vi "3.1.vi"(8 "error in (no error)":errorcluster, 10 "String":string) -> (0 "error out":errorcluster, 2 "Numeric":i32)   [LabVIEW 2017]
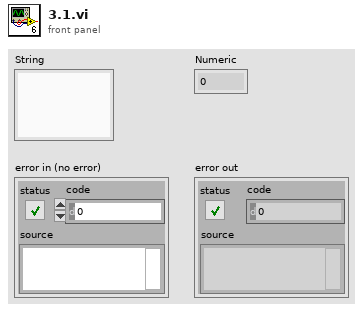
[diagram p1: front panel]
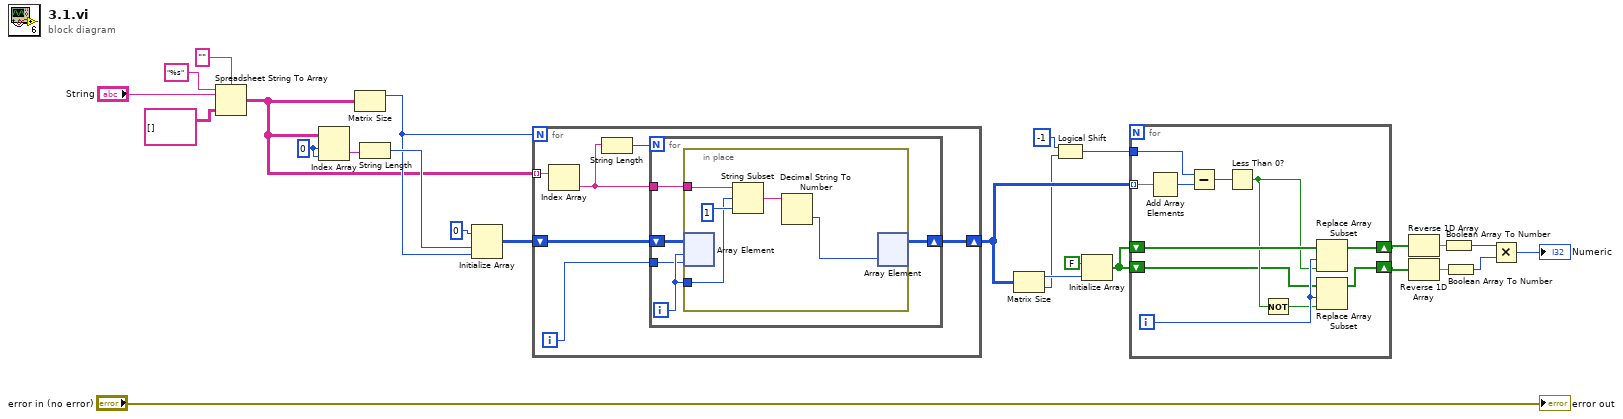
[diagram p0: block diagram]
diagram:
  w22 = 0 ("index (row)")
  n1 = Spreadsheet String To Array(delimiter (Tab)="", format string="%s", spreadsheet string="String", array type (2D Dbl)=string[][] []) -> (array=w15:string[][])
  n2 = Index Array(array=w15, index (row)=w22, index (col)=w22) -> (element=w21:string)
  n3 = Matrix Size(0:w15) -> (1:w16:i32)  [unwired: 1 out]
  n4 = String Length(string=w21) -> (length=w18:i32)
  n5 = Initialize Array(0 ("element"), w18, w16) -> (w17:i32[][])
  n6 = for {
    N: w16 -> [_]
    tunnel: w15 -> [w30] mode=indexing
    shift-right: [w27] -> w13
    shift-left: w17 -> [w32]
    i -> [w31]
    n7 = Index Array(array=w30) -> (element=w29:string)  [unwired: 1 in]
    n8 = String Length(string=w29) -> (length=w28:i32)
    n9 = for {
      N: w28 -> [_]
      shift-right: [w35] -> w27
      shift-left: w32 -> [w37]
      tunnel: w31 -> [w33]
      tunnel: w29 -> [w36]
      i -> [w34]
      n10 = in-place {
        in-place-border: w36 -> [w41]
        in-place-border: w34 -> [w40]
        n11 = in-place-array #1(w37, w34, w33) -> ()  [unwired: 1 out]
        n12 = String Subset(string=w41, offset (0)=w40, length (rest)=1 ("length (rest)")) -> (substring=w39:string)
        n13 = Decimal String To Number(string=w39) -> (number=w38:i32)  [unwired: 2 in, 1 out]
        n14 = in-place-array #1(w38) -> (w35:i32[][])  [unwired: 2 out]
      }
    }
  }
  n15 = Matrix Size(0:w13) -> (1:w12:i32, 2:w9:i32)
  n16 = Logical Shift(y=i16 -1, x=w9) -> (x << y=w8:i32)
  n17 = Initialize Array(FALSE, w12) -> (w11:bool[])
  n18 = for {
    tunnel: w13 -> [w53] mode=indexing
    tunnel: w8 -> [w51]
    shift-right: [w43] -> w5
    shift-left: w11 -> [w49]
    shift-right: [w44] -> w4
    shift-left: w11 -> [w45]
    i -> [w48]
    n19 = Add Array Elements(numeric array=w53) -> (sum=w52:i32)
    n20 = Subtract(x=w51, y=w52) -> (x-y=w50:i32)
    n21 = Less Than 0?(x=w50) -> (x < 0?=w47:bool)
    n22 = Not(x=w47) -> (.not. x?=w46:bool)
    n23 = Replace Array Subset(array=w49, new element=w47, index=w48) -> (w43:bool[])
    n24 = Replace Array Subset(array=w45, new element=w46, index=w48) -> (w44:bool[])
  }
  n25 = Reverse 1D Array(array=w5) -> (reversed array=w7:bool[])
  n26 = Reverse 1D Array(array=w4) -> (reversed array=w6:bool[])
  n27 = Boolean Array To Number(Boolean array=w7) -> (number=w2:u32)
  n28 = Boolean Array To Number(Boolean array=w6) -> (number=w3:u32)
  n29 = Multiply(x=w2, y=w3) -> (x*y=→"Numeric":u32)
  "error out" <- "error in (no error)"
